vi "read_LaserFireThreshold.vi"() -> ()   [LabVIEW 2014]
panel:
  out "Fire Threshold":dbl
  in  "Num Bytes to Fetch (64)":u8=64 min=1
  out "dup Aardvark Handle":i32
  out "error out":errorcluster
  in  "error in (no error)":errorcluster
  in  "Address (0x50)":u16=80 max=1023 format="%.0x"
  in  "Aardvark Handle":i32 min=0
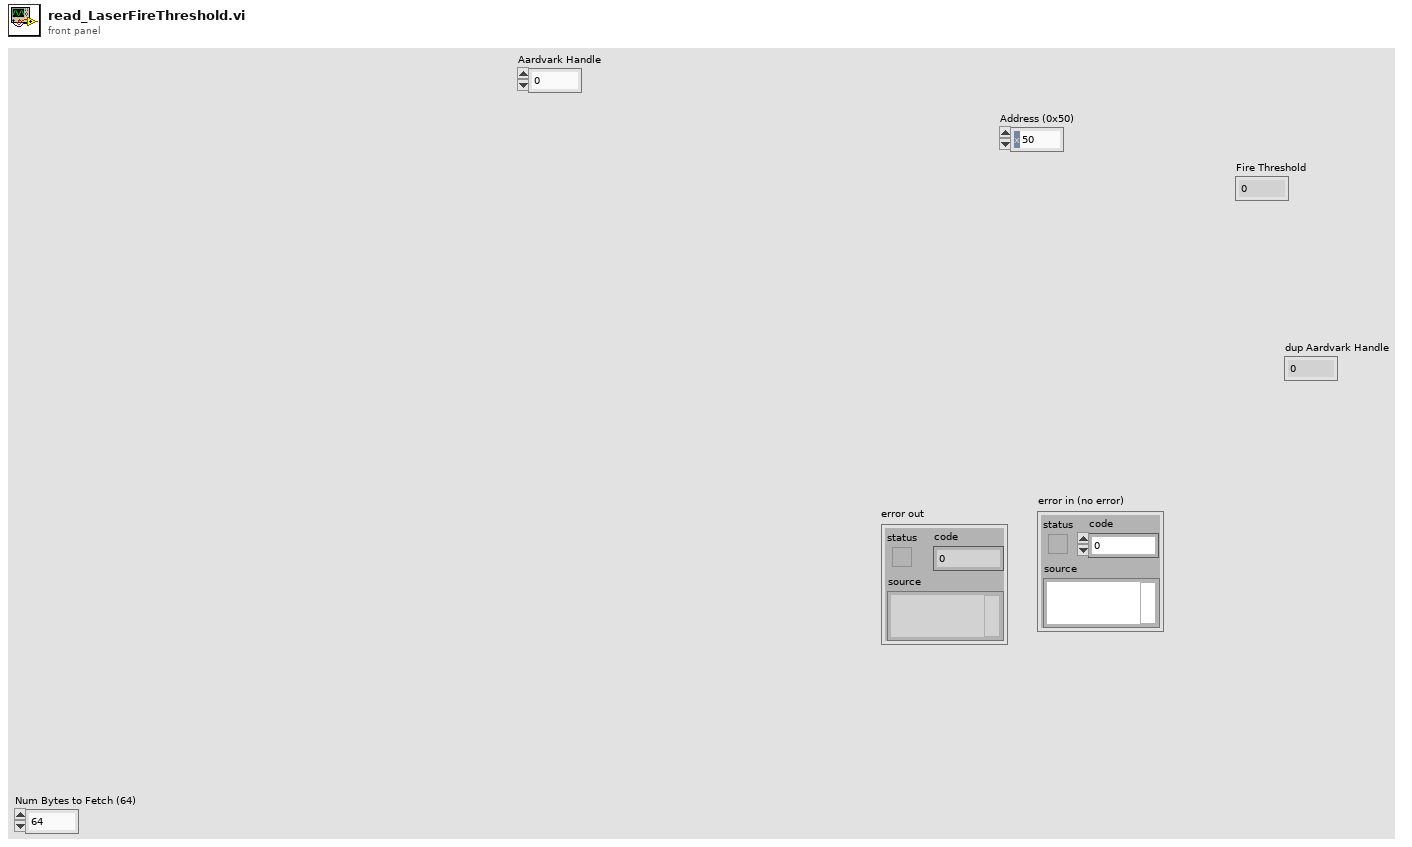
[diagram p1: front panel]
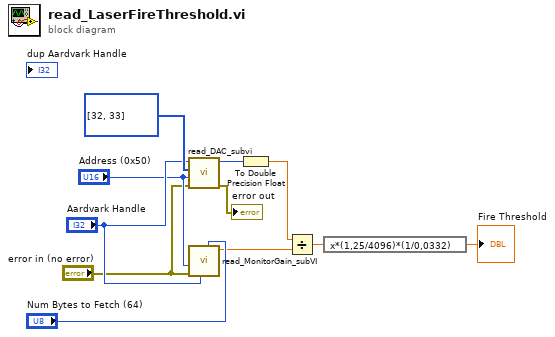
[diagram p0: block diagram]
diagram:
  n1 = call "read_DAC_subvi.vi"("error in (no error)"="error in (no error)", "Address (0x50) in"="Address (0x50)", "DAC_ADD"=u8[] [32, 33], "Aardvark Handle in"="Aardvark Handle") -> ("error out"=→"error out":errorcluster, "DAC Val"=w5:u16)  [unwired: 6 in]
  n2 = call "read_MonitorGain_subVI.vi"("Num Bytes to Fetch (64) in"="Num Bytes to Fetch (64)", "Aardvark Handle in"="Aardvark Handle", "error in (no error)"="error in (no error)", "Address (0x50) in"="Address (0x50)") -> ("Gain"=w3:dbl)  [unwired: 7 in]
  n3 = To Double Precision Float(number=w5) -> (double precision float=w4:dbl)
  n4 = Divide(x=w4, y=w3) -> (x/y=w2:dbl)
  n5 = expression code="x*(1,25/4096)*(1/0,0332)"(w2) -> (→"Fire Threshold":dbl)
